vi "ExpGet.vi"(8 "error in":errorcluster, 11 "ExpID":string) -> (0 "error out":errorcluster, 3 "Exp Info":T1={"ExposeInfo"={"CSCom"=refnum, "URL"="", "Events Category"="", "ID"="", "SRefID"=""}, "ExpID"="[noexp]", "ExperimentFilename"="", "Caller Keep Alive"=refnum})   [LabVIEW 2017]
uses:
  ExperimentInfo.ctl
  Expose/Labview/Core/ExposeInfo.ctl
  C:/Code/CMCryoSysCode/Expose/COM/CSCom/CSCom/bin/Release/CSCom.dll
  Expose/COM/CSCom/CSCom/bin/Release/CSCom.dll
  ExpGlobals.vi
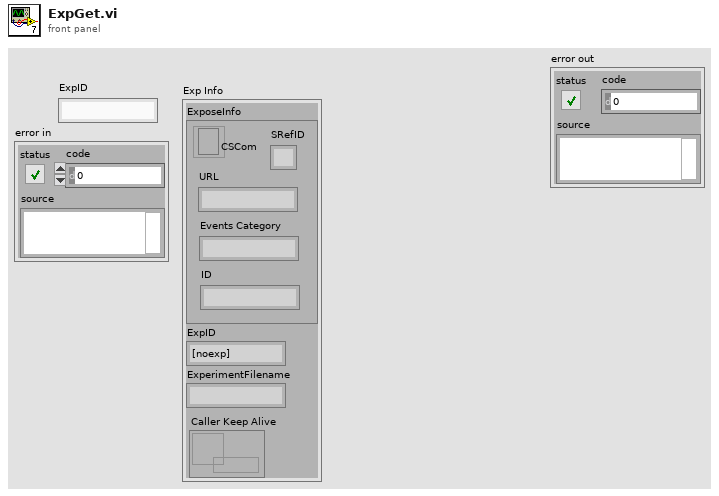
[diagram p1: front panel]
types:
  T1 = typedef "ExperimentInfo.ctl" = cluster{"ExposeInfo":T2, "ExpID":string, "ExperimentFilename":string, "Caller Keep Alive":refnum<data-value>}
  T2 = typedef "ExposeInfo.ctl" = cluster{"CSCom":refnum<k24>, "URL":string, "Events Category":string, "ID":string, "SRefID":string}
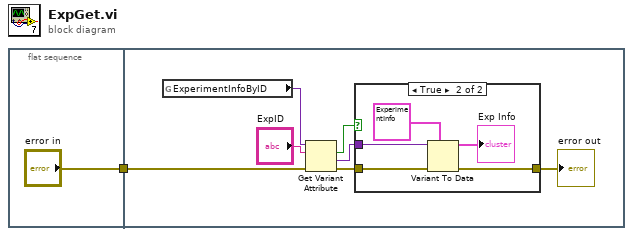
[diagram p0: block diagram]
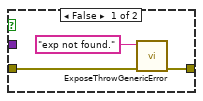
[diagram p2: hidden frame]
diagram:
  n1 = flat-sequence {
    tunnel: ["error in"] -> w1
    tunnel: w1 -> [w5]
    frame #0 {
    }
    frame #1 {
      n2 = global read "ExpGlobals.vi" "ExperimentInfoByID"() -> (w6:variant)
      n3 = Get Variant Attribute(Variant=w6, name="ExpID", error in=w5) -> (found=w8:bool, value=w9:variant, error out=w4:errorcluster)  [unwired: 1 in, 1 out]
      n4 = case shown="True" w8 {
        tunnel: w9 -> [_ w17]
        tunnel: w4 -> [w11 w14]
        tunnel: [w10 w13] -> w3
        frame False {
          n5 = call "ExposeThrowGenericError.vi"("error in (no error)"=w11, "TheError"="exp not found.") -> ("error out"=w10:errorcluster)  [unwired: 9 in]
        }
        frame True {
          n6 = Variant To Data(error in=w14, type=T1 {"ExposeInfo"={"CSCom"=refnum, "URL"="", "Events Category"="", "ID"="", "SRefID"=""}, "ExpID"="[noexp]", "ExperimentFilename"="", "Caller Keep Alive"=refnum} ("Exp Info"), Variant=w17) -> (data=→"Exp Info":T1, error out=w13:errorcluster)
        }
      }
      "error out" <- w3
    }
  }
